vi "Convert to CBOR.vi"(8 "error in (no error)":errorcluster, 10 "CBOR HEX (empty)":string, 11 "JSON Object":string) -> (0 "error out":errorcluster, 3 "CBOR HEX":string)   [LabVIEW 2020, in "CBOR.lvlib"]
doc: "Convert JSON Structure into CBOR Hex recursively"
uses:
  CBOR.lvlib
  Controls/Structure Options.ctl
  <vilib>/JDP Science/JSONtext/JSONtext.lvlib
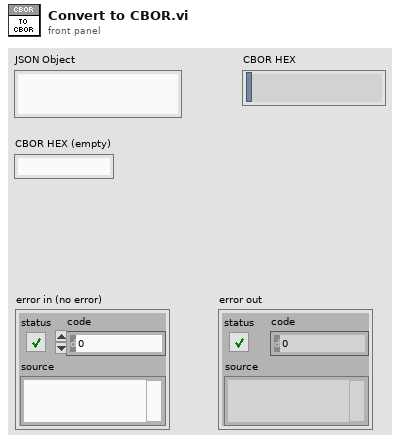
[diagram p1: front panel]
types:
  T1 = typedef "JSONtext.lvlib/JSON Value Type.ctl" = enum16{"Not a JSON Value", "JSON Object", "JSON Array", "String", "Number", "true", "false", "null"}
  T2 = typedef "CBOR.lvlib/Structure Options.ctl" = enum16{"Map", "Text", "Array", "Integer", "Float"}
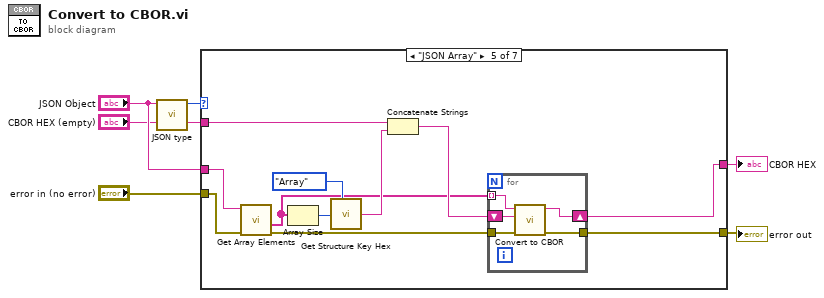
[diagram p0: block diagram]
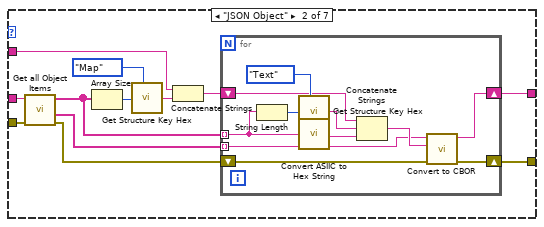
[diagram p3: hidden frame]
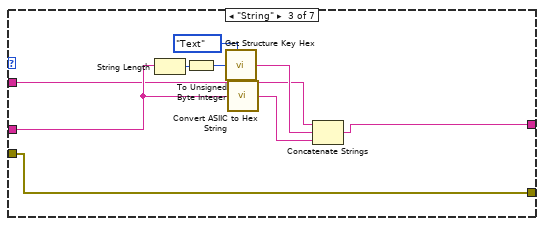
[diagram p4: hidden frame]
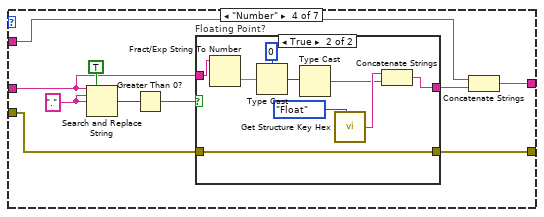
[diagram p5: hidden frame]
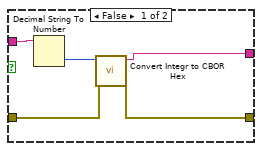
[diagram p6: hidden frame]
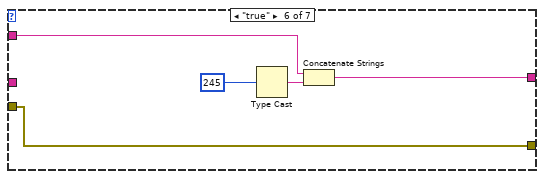
[diagram p7: hidden frame]
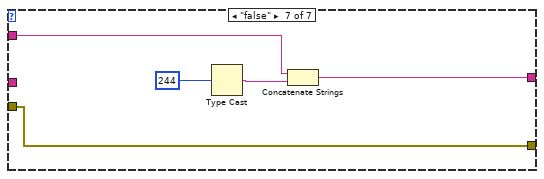
[diagram p8: hidden frame]
diagram:
  n1 = call <vilib>:"JSON type.vi"("JSON"="JSON Object") -> ("JSON Value Type"=w6:T1)  [unwired: 9 in, 1 out]
  n2 = case shown="\"JSON Array\"" w6 {
    tunnel: "JSON Object" -> [_ w20 w35 w46 w74 _ _]
    tunnel: "error in (no error)" -> [w7 w19 w33 w42 w70 w85 w90]
    tunnel: "CBOR HEX (empty)" -> [w8 w15 w34 w44 w75 w84 w89]
    tunnel: [w8 w10 w36 w43 w65 w83 w88] -> w2
    tunnel: [w7 w9 w33 w41 w66 w85 w90] -> w1
    frame "Not a JSON Value", Default {
    }
    frame "JSON Object" {
      n3 = call <vilib>:"Get all Object Items.vi"("error in (no error)"=w19, "JSON"=w20) -> ("error out"=w11:errorcluster, "<JSON>"=w13:string[], "Item Names"=w12:string[])  [unwired: 6 in, 1 out]
      n4 = Array Size(array=w12) -> (size(s)=w18:i32)
      n5 = call "Get Structure Key Hex.vi"("Struct Options"=Structure_Options."Map", "# Struct Elements"=w18) -> ("Key"=w16:string)  [unwired: 7 in]
      n6 = Concatenate Strings(w15, w16) -> (w14:string)
      n7 = for {
        shift-right: [w22] -> w10
        shift-left: w14 -> [w28]
        tunnel: w13 -> [w24] mode=indexing
        tunnel: w12 -> [w30] mode=indexing
        shift-right: [w21] -> w9
        shift-left: w11 -> [w23]
        n8 = String Length(string=w30) -> (length=w31:i32)
        n9 = call "Get Structure Key Hex.vi"("Struct Options"=Structure_Options."Text", "# Struct Elements"=w31) -> ("Key"=w27:string)  [unwired: 7 in]
        n10 = call "Convert ASIIC to Hex String.vi"("String"=w30) -> ("Hex String"=w26:string)  [unwired: 4 in]
        n11 = Concatenate Strings(w28, w27, w26) -> (w25:string)
        n12 = call "Convert to CBOR.vi"("error in (no error)"=w23, "CBOR HEX (empty)"=w25, "JSON Object"=w24) -> ("error out"=w21:errorcluster, "CBOR HEX"=w22:string)  [unwired: 7 in]
      }
    }
    frame "String" {
      n13 = String Length(string=w35) -> (length=w40:i32)
      n14 = To Unsigned Byte Integer(number=w40) -> (unsigned 8bit integer=w32:u8)
      n15 = call "Get Structure Key Hex.vi"("Struct Options"=Structure_Options."Text", "# Struct Elements"=w32) -> ("Key"=w38:string)  [unwired: 7 in]
      n16 = call "Convert ASIIC to Hex String.vi"("String"=w35) -> ("Hex String"=w37:string)  [unwired: 4 in]
      n17 = Concatenate Strings(w34, w38, w37) -> (w36:string)
    }
    frame "Number" {
      w49 = "." ("search string")
      n18 = Search and Replace String(replace all?=TRUE ("replace all? (F)"), input string=w46, search string=w49, replace string=w49) -> (number of replacements=w50:i32)  [unwired: 4 in, 3 out]
      n19 = Greater Than 0?(x=w50) -> (x > 0?=w47:bool)
      n20 = case "Floating Point?" shown="True" w47 {
        tunnel: w46 -> [w55 w64]
        tunnel: [w53 w60] -> w45
        tunnel: w42 -> [w52 w58]
        tunnel: [w51 w58] -> w41
        frame False {
          n21 = Decimal String To Number(string=w55) -> (number=w54:i32)  [unwired: 2 in, 1 out]
          n22 = call "Convert Integr to CBOR Hex.vi"("error in (no error)"=w52, "Integer"=w54) -> ("error out"=w51:errorcluster, "CBOR Hex"=w53:string)  [unwired: 8 in]
        }
        frame True {
          n23 = Fract/Exp String To Number(string=w64) -> (number=w63:dbl)  [unwired: 3 in, 1 out]
          n24 = Type Cast(type=u64 0, x=w63) -> (*(type *) &x=w57:u64)
          n25 = Type Cast(x=w57) -> (*(type *) &x=w56:string)  [unwired: 1 in]
          n26 = call "Get Structure Key Hex.vi"("Struct Options"=Structure_Options."Float") -> ("Key"=w59:string)  [unwired: 8 in]
          n27 = Concatenate Strings(w59, w56) -> (w60:string)
        }
      }
      n28 = Concatenate Strings(w44, w45) -> (w43:string)
    }
    frame "JSON Array" {
      n29 = call <vilib>:"Get Array Elements.vi"("error in (no error)"=w70, "JSON"=w74) -> ("error out"=w67:errorcluster, "<JSON>"=w68:string[])  [unwired: 7 in, 1 out]
      n30 = Array Size(array=w68) -> (size(s)=w72:i32)
      n31 = call "Get Structure Key Hex.vi"("Struct Options"=Structure_Options."Array", "# Struct Elements"=w72) -> ("Key"=w71:string)  [unwired: 7 in]
      n32 = Concatenate Strings(w75, w71) -> (w69:string)
      n33 = for {
        tunnel: w68 -> [w76] mode=indexing
        tunnel: w67 -> [w80]
        shift-right: [w79] -> w65
        shift-left: w69 -> [w77]
        tunnel: [w78] -> w66
        n34 = call "Convert to CBOR.vi"("error in (no error)"=w80, "CBOR HEX (empty)"=w77, "JSON Object"=w76) -> ("error out"=w78:errorcluster, "CBOR HEX"=w79:string)  [unwired: 7 in]
      }
    }
    frame "true" {
      n35 = Type Cast(x=u8 245) -> (*(type *) &x=w82:string)  [unwired: 1 in]
      n36 = Concatenate Strings(w84, w82) -> (w83:string)
    }
    frame "false" {
      n37 = Type Cast(x=u8 244) -> (*(type *) &x=w86:string)  [unwired: 1 in]
      n38 = Concatenate Strings(w89, w86) -> (w88:string)
    }
  }
  "CBOR HEX" <- w2
  "error out" <- w1
